vi "Value (U16).vi"(10 "error in (no error)":errorcluster, 11 "Config Element in":refnum<class "Config Element.lvclass">) -> (2 "error out":errorcluster, 3 "U16 Value":u16)   [LabVIEW 2020, in "CDM-Config.lvlib" / "Config Element.lvclass"]
uses:
  Config Element.lvclass
  Config Element.lvclass/Config Element.ctl
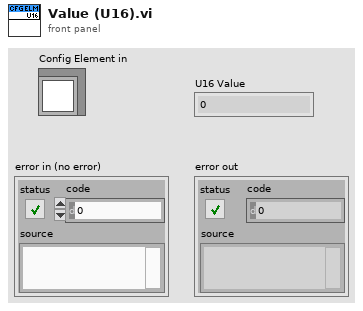
[diagram p1: front panel]
types:
  T1 = typedef "CDM-Config.lvlib/Config Element.lvclass/Ref Data.ctl" = cluster{"Node Info":T2, "Owner":refnum<class>, "Changed":bool, "Name":string, "Meta Data":T3[], "Array":bool, "Value Type":T4, "Value":variant}
  T2 = typedef "CDM-Config.lvlib/Node Info.ctl" = cluster{"Index":i32, "Parent":i32, "Children":i32[]}
  T3 = typedef "CDM-Config.lvlib/Meta Data.ctl" = cluster{"Name":string, "Value":string}
  T4 = typedef "CDM-Config.lvlib/Value Type.ctl" = enum16{"String", "Number", "Bool", "Object", "Array"}
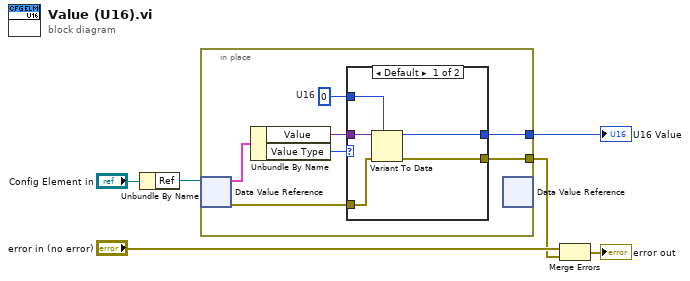
[diagram p0: block diagram]
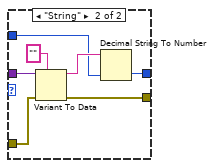
[diagram p2: hidden frame]
diagram:
  n1 = Unbundle By Name("Config Element in") -> ("Ref"=w3:refnum<data-value>)
  n2 = in-place {
    in-place-border: [w9] -> w2
    in-place-border: [w8] -> w1
    w7 = u16 0  # U16
    n3 = in-place-dvr #1(w3) -> (w13:T1, w12:errorcluster)
    n4 = Unbundle By Name(w13) -> ("Value"=w10:variant, "Value Type"=w11:T4)
    n5 = case shown="Default" w11 {
      tunnel: w12 -> [w16 w20]
      tunnel: w10 -> [w18 w25]
      tunnel: [w17 w22] -> w9
      tunnel: [w15 w21] -> w8
      tunnel: w7 -> [w14 w19]
      frame Default {
        n6 = Variant To Data(error in=w16, type=w14, Variant=w18) -> (data=w17:u16, error out=w15:errorcluster)
      }
      frame "String" {
        n7 = Variant To Data(error in=w20, type="", Variant=w25) -> (data=w23:string, error out=w21:errorcluster)
        n8 = Decimal String To Number(string=w23, default (0L)=w19) -> (number=w22:u16)  [unwired: 1 in, 1 out]
      }
    }
    n9 = in-place-dvr #1() -> ()  [unwired: 1 in, 2 out]
  }
  "U16 Value" <- w2
  n10 = Merge Errors("error in (no error)", w1) -> (→"error out":errorcluster)
